vi "ATF-RT Con FGV.vi"(0 "Storage rt con":bool, 1 "Enum":enum16{"Read", "Write"}(ring), 5 "Storage IP":string, 7 "Pumb rt con":bool, 9 "Pump IP":string, 11 "error in":errorcluster) -> (4 "Stoarge rt con R":bool, 6 "Storage IP  R":string, 8 "Pumb rt con R":bool, 10 "Pump IP R":string, 15 "error out":errorcluster)   [LabVIEW 2022 SP3]
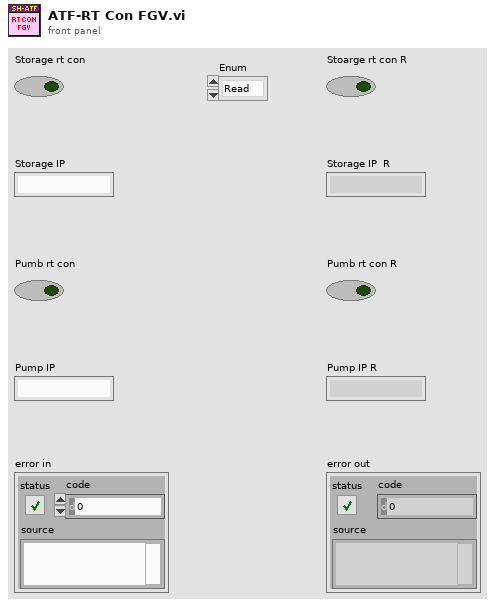
[diagram p1: front panel]
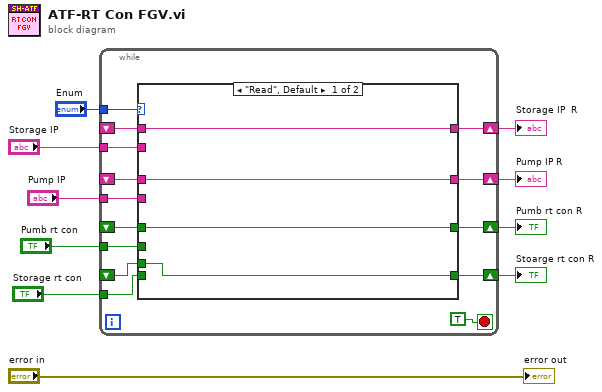
[diagram p0: block diagram]
diagram:
  n1 = while {
    tunnel: "Enum" -> [w24]
    tunnel: "Storage rt con" -> [w22]
    shift-right: [w21] -> w7
    shift-left: _ -> [w20]
    tunnel: "Pumb rt con" -> [w18]
    shift-right: [w19] -> w6
    shift-left: _ -> [w17]
    tunnel: "Pump IP" -> [w16]
    shift-right: [w15] -> w3
    shift-left: _ -> [w14]
    tunnel: "Storage IP" -> [w13]
    shift-right: [w12] -> w1
    shift-left: _ -> [w11]
    stop <- TRUE stop-if-true
    n2 = case shown="\"Read\", Default" w24 {
      tunnel: w22 -> [_ w32]
      tunnel: [w28 w32] -> w21
      tunnel: w20 -> [w28 _]
      tunnel: [w27 w31] -> w19
      tunnel: w18 -> [_ w31]
      tunnel: w17 -> [w27 _]
      tunnel: [w26 w30] -> w15
      tunnel: w16 -> [_ w30]
      tunnel: w14 -> [w26 _]
      tunnel: [w25 w29] -> w12
      tunnel: w13 -> [_ w29]
      tunnel: w11 -> [w25 _]
      frame "Read", Default {
      }
      frame "Write" {
      }
    }
  }
  "Stoarge rt con R" <- w7
  "Pumb rt con R" <- w6
  "Pump IP R" <- w3
  "Storage IP  R" <- w1
  "error out" <- "error in"
